vi "make_synth_array (SubVI).vi"(11 "Synth settings:":T1) -> (1 "DC array":ext[](array[numeric]), 2 "Freq array":ext[](array[numeric]), 3 "AC array":ext[](array[numeric]))   [LabVIEW 2014]
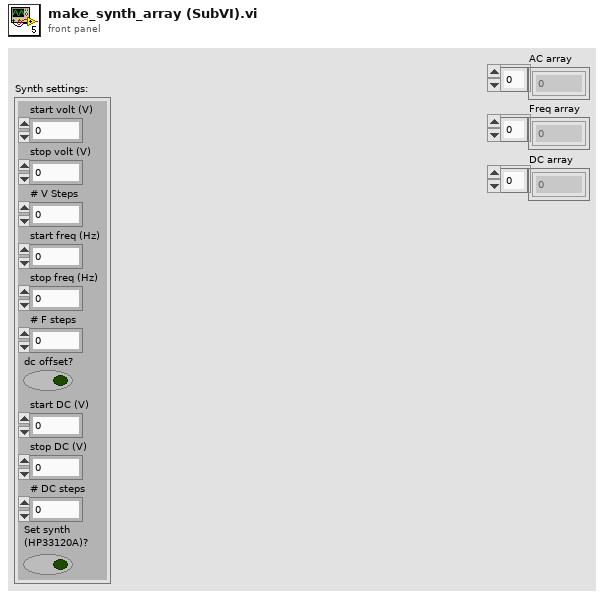
[diagram p1: front panel]
types:
  T1 = cluster{"start volt (V)":ext, "stop volt (V) ":ext, "# V Steps":i32, "start freq (Hz)":ext, "stop freq (Hz) ":ext, "# F steps":i32, "dc offset?":bool, "start DC (V)":ext, "stop DC (V)":ext, "# DC steps ":i32, "Set synth\n(HP33120A)?":bool}
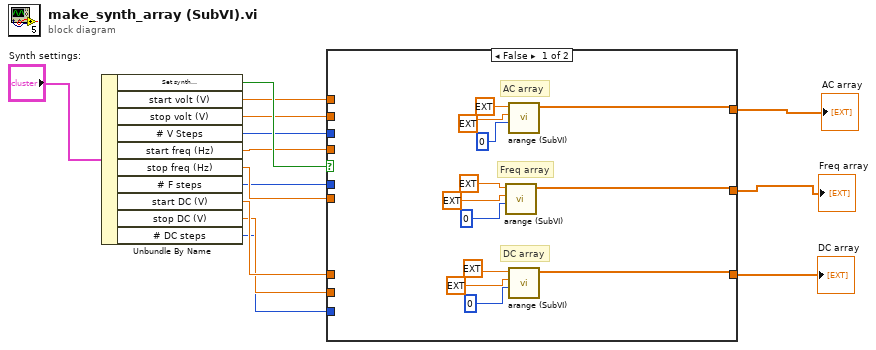
[diagram p0: block diagram]
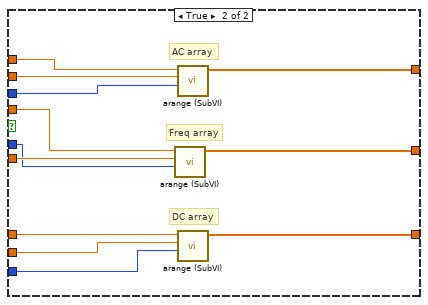
[diagram p2: hidden frame]
diagram:
  n1 = Unbundle By Name("Synth settings:") -> ("Set synth\n(HP33120A)?"=w13:bool, "start volt (V)"=w12:ext, "stop volt (V)"=w11:ext, "# V Steps"=w10:i32, "start freq (Hz)"=w9:ext, "stop freq (Hz)"=w8:ext, "# F steps"=w7:i32, "start DC (V)"=w6:ext, "stop DC (V)"=w5:ext, "# DC steps"=w4:i32)
  n2 = case shown="False" w13 {
    tunnel: w12 -> [_ w38]
    tunnel: w11 -> [_ w37]
    tunnel: w10 -> [_ w36]
    tunnel: w9 -> [_ w35]
    tunnel: w8 -> [_ w34]
    tunnel: w7 -> [_ w33]
    tunnel: w6 -> [_ w32]
    tunnel: w5 -> [_ w31]
    tunnel: w4 -> [_ w30]
    tunnel: [w17 w29] -> w3
    tunnel: [w16 w28] -> w2
    tunnel: [w15 w27] -> w1
    frame False {
      # "DC array"
      # "Freq array"
      # "AC array"
      n3 = call "arange (SubVI).vi"("# Steps"=0, "stop"=ext 0.0, "start"=ext 0.0) -> ("Array"=w16:ext[])  [unwired: 8 in]
      n4 = call "arange (SubVI).vi"("# Steps"=0, "stop"=ext 0.0, "start"=ext 0.0) -> ("Array"=w17:ext[])  [unwired: 8 in]
      n5 = call "arange (SubVI).vi"("# Steps"=0, "stop"=ext 0.0, "start"=ext 0.0) -> ("Array"=w15:ext[])  [unwired: 8 in]
    }
    frame True {
      # "DC array"
      # "Freq array"
      # "AC array"
      n6 = call "arange (SubVI).vi"("# Steps"=w33, "stop"=w34, "start"=w35) -> ("Array"=w28:ext[])  [unwired: 8 in]
      n7 = call "arange (SubVI).vi"("# Steps"=w36, "stop"=w37, "start"=w38) -> ("Array"=w29:ext[])  [unwired: 8 in]
      n8 = call "arange (SubVI).vi"("# Steps"=w30, "stop"=w31, "start"=w32) -> ("Array"=w27:ext[])  [unwired: 8 in]
    }
  }
  "AC array" <- w3
  "Freq array" <- w2
  "DC array" <- w1
